vi "demo_Set Icon Text.vi"(11 "Stop Demo":refnum<user-event>) -> ()   [LabVIEW 2020]
panel:
  # "Ctrl-K"
  # "LabVIEW 2020 - Set Icon Text from Quick Drop\n\nYou can use the Ctrl-K shortcut in Quick Drop to apply a simple text-based icon to your VI, without having to launch the Icon Editor."
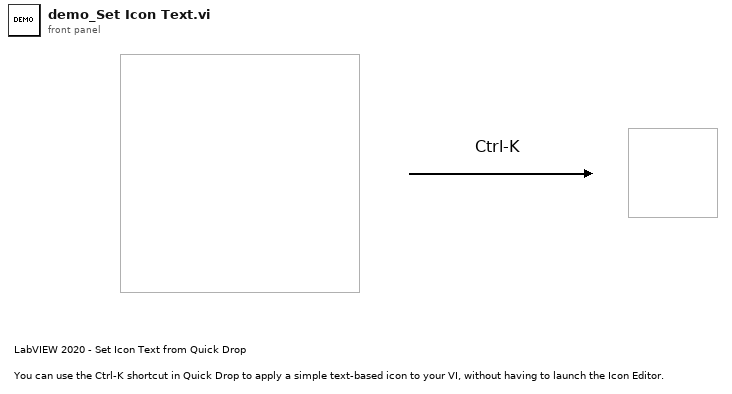
[diagram p1: front panel]
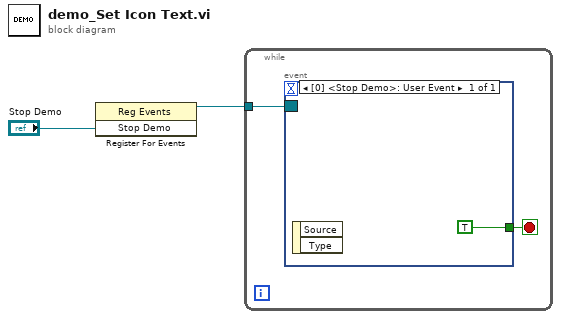
[diagram p0: block diagram]
diagram:
  n1 = register-events("Stop Demo") -> (reference out=w1:refnum<event-registration>)  [unwired: 2 in, 1 out]
  n2 = while {
    tunnel: w1 -> [w4]
    stop <- w3 stop-if-true
    n3 = event shown="[0] <Stop Demo>: User Event" {
      selector: w4 -> [_]
      dyn-events: _ -> [_]
      timeout: _ -> [_]
      tunnel: [TRUE] -> w3
      event User Event {
        n4 = event-data() -> ()  [unwired: 1 in, 2 out]
      }
    }
  }
